vi "SenCMD.vi"() -> ()   [LabVIEW 2011]
panel:
  out "error out 2":errorcluster
  out "error out":errorcluster
  in  "Numeric":i32
  in  "stop":bool
  # "0 \n1 Exit\n2 Set Rea\n3 set oad"
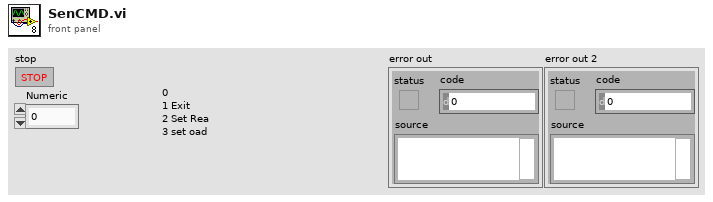
[diagram p1: front panel]
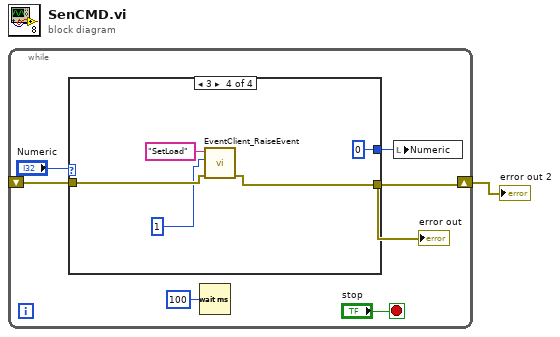
[diagram p0: block diagram]
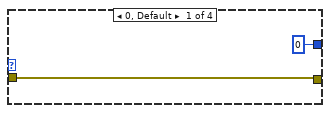
[diagram p2: hidden frame]
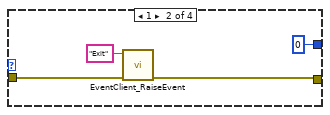
[diagram p3: hidden frame]
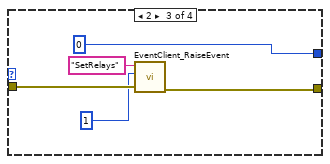
[diagram p4: hidden frame]
diagram:
  n1 = while {
    shift-right: [w4] -> w1
    shift-left: _ -> [w5]
    stop <- "stop" stop-if-true
    n2 = case shown="3" "Numeric" {
      tunnel: w5 -> [w9 w12 w17 w22]
      tunnel: [w9 w11 w16 w21] -> w4
      tunnel: [0 ("Numeric") 0 ("Numeric") 0 ("Numeric") 0 ("Numeric")] -> w2
      frame 0, Default {
      }
      frame 1 {
        n3 = call "EventClient_RaiseEvent.vi"("error in (no error)"=w12, "Event"="Exit") -> ("error out"=w11:errorcluster)  [unwired: 9 in]
      }
      frame 2 {
        n4 = call "EventClient_RaiseEvent.vi"("error in (no error)"=w17, "Data"=u16 1 ("Numeric"), "Event"="SetRelays") -> ("error out"=w16:errorcluster)  [unwired: 8 in]
      }
      frame 3 {
        n5 = call "EventClient_RaiseEvent.vi"("error in (no error)"=w22, "Data"=u16 1 ("Numeric"), "Event"="SetLoad") -> ("error out"=w21:errorcluster)  [unwired: 8 in]
      }
    }
    "error out" <- w4
    n6 = Wait (ms)(milliseconds to wait=u32 100) -> ()  [unwired: 1 out]
    n7 = local write "Numeric"(w2) -> ()
  }
  "error out 2" <- w1
